vi "SUB_WIH_SFCS_SendResult_NoAsk.vi"(1 "ErrorCode":string, 2 "PASS_Fail (1/0)":i8) -> (0 "Sent OK ?":bool)   [LabVIEW 2011]
uses:
  Instance           6 33Saved   SUB_SFCS_SendResult_NoAsk .vi
  Instance           4 33Saved   SUB_SFCS_SendResult_NoAsk .vi
  Instance           2 33Saved   SUB_SFCS_SendResult_NoAsk .vi
  Instance           7 33Saved   SUB_SFCS_SendResult_NoAsk .vi
  Instance           8 33Saved   SUB_SFCS_SendResult_NoAsk .vi
  Instance           9 33Saved   SUB_SFCS_SendResult_NoAsk .vi
  Instance          10 33Saved   SUB_SFCS_SendResult_NoAsk .vi
panel:
  out "SFCS System Enable":string
  out "OperatorID":string
  out "Line":string
  out "SN":string
  out "Station":string
  out "STAGE":string
  out "SFCS_IP":string
  # "Send Result SFCS_Complete"
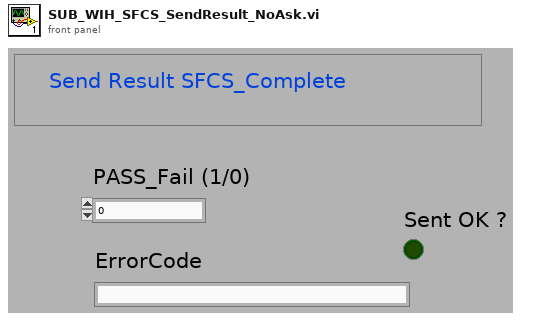
[diagram p1: front panel]
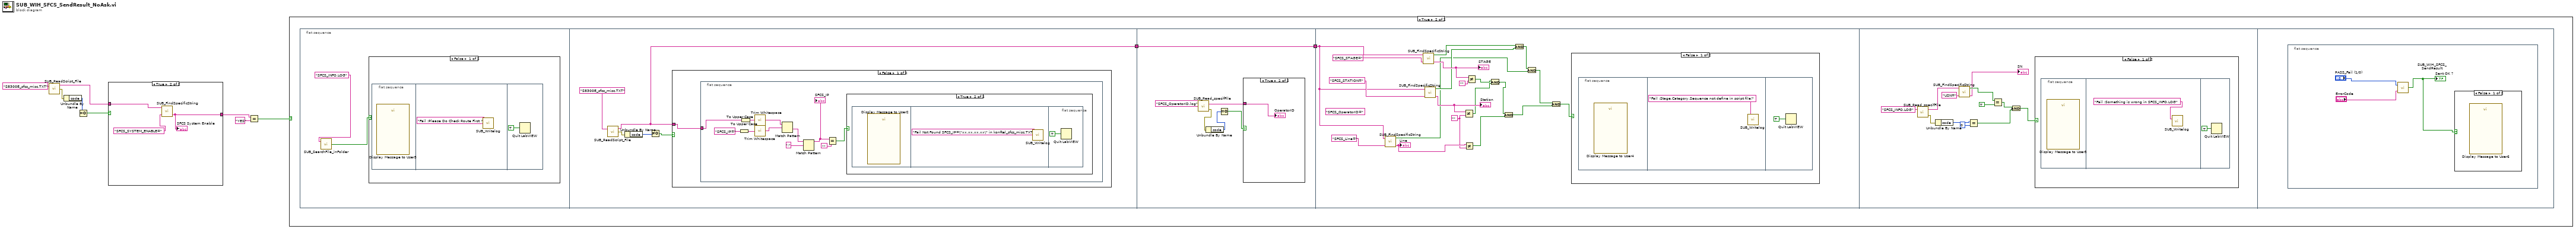
[diagram p0: block diagram]
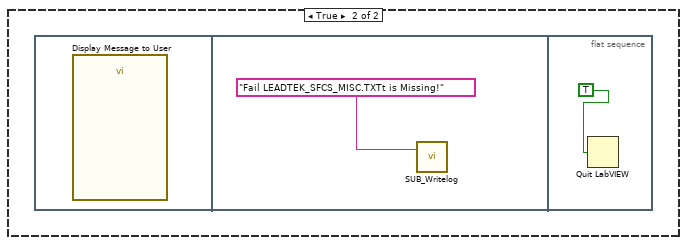
[diagram p5: hidden frame]
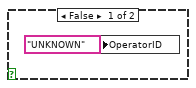
[diagram p6: hidden frame]
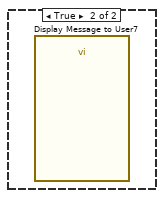
[diagram p9: hidden frame]
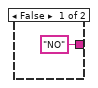
[diagram p10: hidden frame]
diagram:
  n1 = call "SUB_ReadScript_File.vi"("Script FileName"="S8300E_sfcs_misc.TXT") -> ("text"=w2:string, "error out"=w8:errorcluster)  [unwired: 1 in, 1 out]
  n2 = Unbundle By Name(w8) -> ("code"=w7:i32)
  n3 = Equal To 0?(x=w7) -> (x = 0?=w6:bool)
  n4 = case shown="True" w6 {
    tunnel: w2 -> [_ w12]
    tunnel: ["NO" ("before \"; \" string") w10] -> w4
    frame False {
    }
    frame True {
      n5 = call "SUB_FindSpecificString.vi"("Find this String"="SFCS_SYSTEM_ENABLE=", "String data"=w12) -> ("before \"; \" string"=w10:string)  [unwired: 2 in, 1 out]
      "SFCS System Enable" <- w10
    }
  }
  n6 = Equal?(x=w4, y="YES") -> (x = y?=w5:bool)
  n7 = case shown="True" w5 {
    frame False {
    }
    frame True {
      n8 = flat-sequence {
        tunnel: [w20] -> w14
        tunnel: w14 -> [w45]
        tunnel: [w45] -> w13
        tunnel: w13 -> [w63]
        frame #0 {
          n9 = call "SUB_SearchFile_inFolder.vi"("Search Filename in Folder"="SFCS_INFO.LOG") -> ("File Existing True/Flase"=w15:bool)  [unwired: 1 in]
          n10 = case shown="False" w15 {
            frame False {
              n11 = flat-sequence {
                frame #0 {
                  n12 = call "Display Message to User3"() -> ()  [unwired: 10 in, 2 out]
                }
                frame #1 {
                  n13 = call "SUB_Writelog.vi"("Pass/Fail"="Fail :Please Do Check Route First !") -> ()  [unwired: 2 in]
                }
                frame #2 {
                  n14 = Quit LabVIEW(quit? (T)=TRUE) -> ()
                }
              }
            }
            frame True {
            }
          }
        }
        frame #1 {
          n15 = call "SUB_ReadScript_File.vi"("Script FileName"="S8300E_sfcs_misc.TXT") -> ("text"=w20:string, "error out"=w23:errorcluster)  [unwired: 1 in, 1 out]
          n16 = Unbundle By Name(w23) -> ("code"=w22:i32)
          n17 = Not Equal To 0?(x=w22) -> (x != 0?=w21:bool)
          n18 = case shown="False" w21 {
            tunnel: w20 -> [w24 _]
            frame False {
              n19 = flat-sequence {
                tunnel: w24 -> [w30]
                frame #0 {
                  n20 = To Upper Case(1:"SFCS_IP=" ("string")) -> (0:w34:string)
                  n21 = To Upper Case(1:w30) -> (0:w35:string)
                  n22 = call <vilib>:"Trim Whitespace.vi"("string"=w34) -> ("trimmed string"=w32:string)  [unwired: 1 in]
                  n23 = call <vilib>:"Trim Whitespace.vi"("string"=w35) -> ("trimmed string"=w31:string)  [unwired: 1 in]
                  n24 = Match Pattern(string=w31, regular expression=w32) -> (after substring=w29:string)  [unwired: 1 in, 3 out]
                  n25 = Match Pattern(string=w29, regular expression=";") -> (before substring=w27:string)  [unwired: 1 in, 3 out]
                  "SFCS_IP" <- w27
                  n26 = Equal?(x=w27, y="") -> (x = y?=w25:bool)
                  n27 = case shown="True" w25 {
                    frame False {
                    }
                    frame True {
                      n28 = flat-sequence {
                        frame #0 {
                          n29 = call "Display Message to User2"() -> ()  [unwired: 10 in, 2 out]
                        }
                        frame #1 {
                          n30 = call "SUB_Writelog.vi"("Pass/Fail"="Fail Not Found SFCS_IP=\"xx.xx.xx.xx\" in konftel_sfcs_misc.TXT !") -> ()  [unwired: 2 in]
                        }
                        frame #2 {
                          n31 = Quit LabVIEW(quit? (T)=TRUE) -> ()
                        }
                      }
                    }
                  }
                }
              }
            }
            frame True {
              n32 = flat-sequence {
                frame #0 {
                  n33 = call "Display Message to User"() -> ()  [unwired: 10 in, 2 out]
                }
                frame #1 {
                  n34 = call "SUB_Writelog.vi"("Pass/Fail"="Fail LEADTEK_SFCS_MISC.TXTt is Missing!") -> ()  [unwired: 2 in]
                }
                frame #2 {
                  n35 = Quit LabVIEW(quit? (T)=TRUE) -> ()
                }
              }
            }
          }
        }
        frame #2 {
          n36 = call "SUB_Read_specifFile.vi"("name or relative path"="SFCS_OperatorID.log") -> ("error out"=w43:errorcluster, "text"=w40:string)  [unwired: 1 in]
          n37 = Unbundle By Name(w43) -> ("code"=w42:i32)
          n38 = Equal To 0?(x=w42) -> (x = 0?=w41:bool)
          n39 = case shown="True" w41 {
            tunnel: w40 -> [_ w47]
            frame False {
              n40 = local write "OperatorID"("UNKNOWN" ("OperatorID")) -> ()
            }
            frame True {
              "OperatorID" <- w47
            }
          }
        }
        frame #3 {
          (unwired) "SFCS_OperatorID="
          w58 = ""
          n41 = call "SUB_FindSpecificString.vi"("Find this String"="SFCS_Line=", "String data"=w63) -> ("before \"; \" string"=w59:string, "Found"=w49:bool)  [unwired: 2 in]
          "Line" <- w59
          n42 = call "SUB_FindSpecificString.vi"("Find this String"="SFCS_STAGE=" ("string"), "String data"=w63) -> ("before \"; \" string"=w61:string, "Found"=w54:bool)  [unwired: 2 in]
          "STAGE" <- w61
          n43 = call "SUB_FindSpecificString.vi"("Find this String"="SFCS_STATION=" ("string"), "String data"=w63) -> ("before \"; \" string"=w60:string, "Found"=w53:bool)  [unwired: 2 in]
          "Station" <- w60
          n44 = Not Equal?(x=w60, y=w58) -> (x != y?=w56:bool)
          n45 = Not Equal?(x=w59, y=w58) -> (x != y?=w48:bool)
          n46 = Not Equal?(x=w61, y="") -> (x != y?=w57:bool)
          n47 = And(x=w57, y=w56) -> (x .and. y?=w55:bool)
          n48 = And(x=w55, y=w48) -> (x .and. y?=w50:bool)
          n49 = And(x=w54, y=w53) -> (x .and. y?=w52:bool)
          n50 = And(x=w52, y=w49) -> (x .and. y?=w51:bool)
          n51 = And(x=w51, y=w50) -> (x .and. y?=w66:bool)
          n52 = case shown="False" w66 {
            frame False {
              n53 = flat-sequence {
                frame #0 {
                  n54 = call "Display Message to User4"() -> ()  [unwired: 10 in, 2 out]
                }
                frame #1 {
                  n55 = call "SUB_Writelog.vi"("Pass/Fail"="Fail :Stage,Category,Sequence not define in script file!") -> ()  [unwired: 2 in]
                }
                frame #2 {
                  n56 = Quit LabVIEW(quit? (T)=TRUE) -> ()
                }
              }
            }
            frame True {
            }
          }
        }
        frame #4 {
          n57 = call "SUB_Read_specifFile.vi"("name or relative path"="SFCS_INFO.LOG") -> ("error out"=w80:errorcluster, "text"=w79:string)  [unwired: 1 in]
          n58 = Unbundle By Name(w80) -> ("code"=w77:i32)
          n59 = call "SUB_FindSpecificString.vi"("Find this String"="USN=", "String data"=w79) -> ("before \"; \" string"=→"SN":string, "Found"=w75:bool)  [unwired: 2 in]
          n60 = Equal?(x=w77, y=0) -> (x = y?=w72:bool)
          n61 = Equal?(x=w75, y=TRUE) -> (x = y?=w73:bool)
          n62 = And(x=w73, y=w72) -> (x .and. y?=w70:bool)
          n63 = case shown="False" w70 {
            frame False {
              n64 = flat-sequence {
                frame #0 {
                  n65 = call "Display Message to User5"() -> ()  [unwired: 10 in, 2 out]
                }
                frame #1 {
                  n66 = call "SUB_Writelog.vi"("Pass/Fail"="Fail :Something is wrong in SFCS_INFO.LOG") -> ()  [unwired: 2 in]
                }
                frame #2 {
                  n67 = Quit LabVIEW(quit? (T)=TRUE) -> ()
                }
              }
            }
            frame True {
            }
          }
        }
        frame #5 {
          n68 = flat-sequence {
            frame #0 {
              n69 = call "SUB_WIH_SFCS_SendResult.vi"("ErrorCode"="ErrorCode", "PASS_Fail (1/0)"="PASS_Fail (1/0)") -> ("Sent OK ?"=w84:bool)
              "Sent OK ?" <- w84
              n70 = case shown="False" w84 {
                frame False {
                  n71 = call "Display Message to User6"() -> ()  [unwired: 10 in, 2 out]
                }
                frame True {
                  n72 = call "Display Message to User7"() -> ()  [unwired: 10 in, 2 out]
                }
              }
            }
          }
        }
      }
    }
  }
